vi "Dynamic Reset SL.vi"(6 "Target resistance (ohm)":dbl, 7 "Step size":dbl, 8 "error in (no error)":errorcluster, 9 "WL voltage ref":refnum<vi>, 10 "SL voltage ref":refnum<vi>, 11 "instrument handle":refnum<k15>) -> (0 "error out":errorcluster, 2 "Final resistance (ohm)":dbl, 3 "instrument handle out":refnum<k15>)   [LabVIEW 2018]
uses:
  Globals.vi
  <instrlib>/niDigital/niDigital.llb/niDigital Burst Pattern (Burst Only).vi
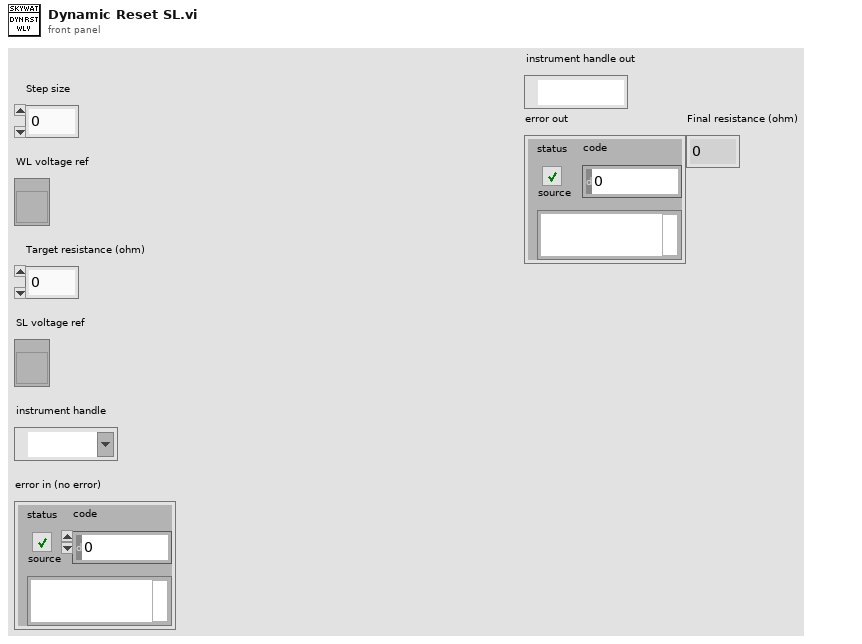
[diagram p1: front panel]
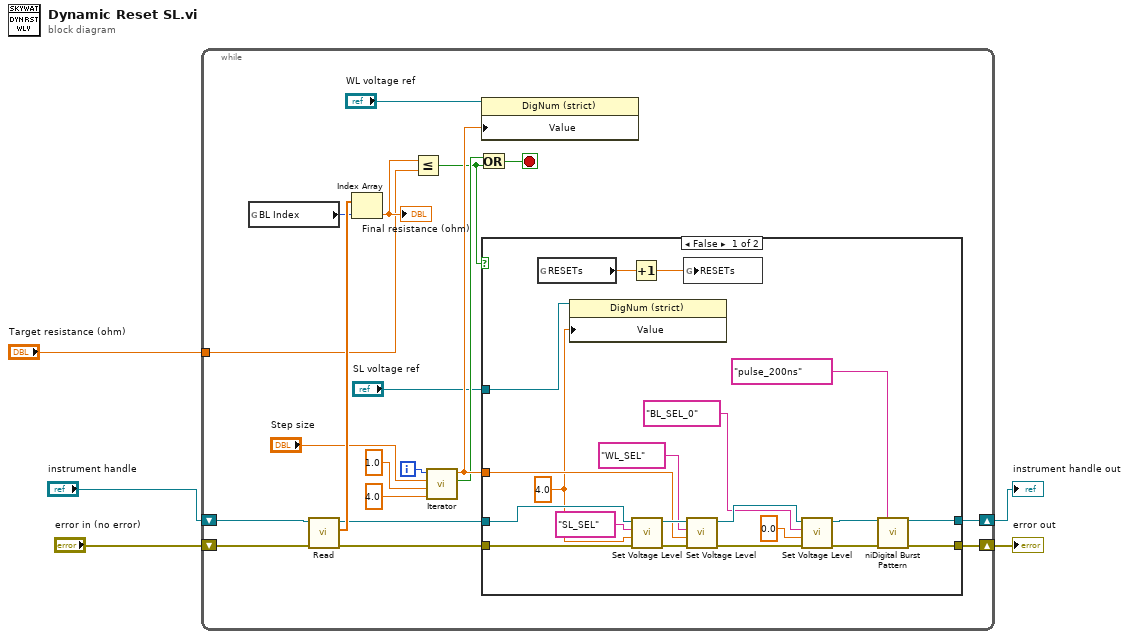
[diagram p0: block diagram]
diagram:
  n1 = while {
    shift-right: [w18] -> w2
    shift-left: "instrument handle" -> [w15]
    shift-right: [w17] -> w1
    shift-left: "error in (no error)" -> [w16]
    tunnel: "Target resistance (ohm)" -> [w9]
    i -> [w24]
    stop <- w12 stop-if-true
    n2 = global read "Globals.vi" "BL Index"() -> (w14:i32)
    n3 = call "Read.vi"("error in (no error)"=w16, "instrument handle"=w15) -> ("error out"=w21:errorcluster, "resistances (ohm)"=w22:dbl[], "instrument handle out"=w20:refnum<k15>)  [unwired: 6 in, 1 out]
    n4 = Index Array(array=w22, index=w14) -> (element=w13:dbl)
    "Final resistance (ohm)" <- w13
    n5 = Less Or Equal?(x=w13, y=w9) -> (x <= y?=w10:bool)
    n6 = call "Iterator.vi"("Final Value"=4.0 ("y"), "Initial Value"=1.0 ("y"), "Step"="Step size", "i"=w24) -> ("End Loop"=w11:bool, "Current Value"=w19:dbl)  [unwired: 6 in]
    n7 = Or(x=w11, y=w10) -> (x .or. y?=w12:bool)
    n8 = property class="DigNum (strict)"(reference="WL voltage ref", "Value"=w19) -> ()  [unwired: 1 in, 2 out]
    n9 = case shown="False" w10 {
      tunnel: [w45 w46] -> w17
      tunnel: [w44 w47] -> w18
      tunnel: w21 -> [w30 w46]
      tunnel: w20 -> [w29 w47]
      tunnel: w19 -> [w27 _]
      tunnel: "SL voltage ref" -> [w28 _]
      frame False {
        w26 = 4.0 ("level (V)")
        n10 = global read "Globals.vi" "RESETs"() -> (w38:dbl)
        n11 = property class="DigNum (strict)"(reference=w28, "Value"=w26) -> ()  [unwired: 1 in, 2 out]
        n12 = Increment(x=w38) -> (x+1=w37:dbl)
        n13 = call "Set Voltage Level.vi"("error in (no error)"=w30, "level (V)"=w26, "channel list"="SL_SEL", "instrument handle"=w29) -> ("error out"=w43:errorcluster, "instrument handle out"=w42:refnum<k15>)  [unwired: 6 in]
        n14 = global write "Globals.vi" "RESETs"(w37) -> ()
        n15 = call "Set Voltage Level.vi"("error in (no error)"=w43, "level (V)"=w27, "channel list"="WL_SEL", "instrument handle"=w42) -> ("error out"=w35:errorcluster, "instrument handle out"=w36:refnum<k15>)  [unwired: 6 in]
        n16 = call "Set Voltage Level.vi"("error in (no error)"=w35, "level (V)"=0.0, "channel list"="BL_SEL_0", "instrument handle"=w36) -> ("error out"=w34:errorcluster, "instrument handle out"=w33:refnum<k15>)  [unwired: 6 in]
        n17 = call-poly <instrlib>:"niDigital Burst Pattern.vi"("instrument handle"=w33, "start label"="pulse_200ns", "error in"=w34) -> ("instrument handle out"=w44:refnum<k15>, "error out"=w45:errorcluster)  [unwired: 11 in]
      }
      frame True {
      }
    }
  }
  "instrument handle out" <- w2
  "error out" <- w1
